vi "GUI_Shutdown.vi"(4 "error in":errorcluster) -> (0 "error out":errorcluster)   [LabVIEW 2015]
doc: "Monitors the manager globals, waiting for a complete shutdown"
panel:
  out "shutting down systems...":dbl(slide) scale=0.0..100.0
  in  "Listbox":i32(listbox)=8
  # "Systems are shutting down.  Mechanical systems are \nreturning to safe configurations. The program will \nterminate automatically when the shutdown is \ncomplete."
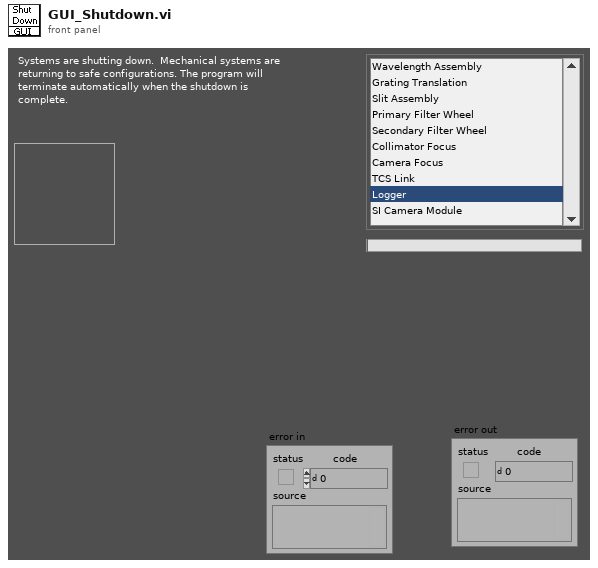
[diagram p1: front panel]
types:
  T1 = cluster{"WL Online":bool, "GT Online":bool, "Slit Online":bool, "F1 Online":bool, "F2 Online":bool, "Coll Online":bool, "CF Online":bool, "TCSLink Online":bool, "Logger Online":bool, "Apogee Online":bool, "TCPServer Online":bool}
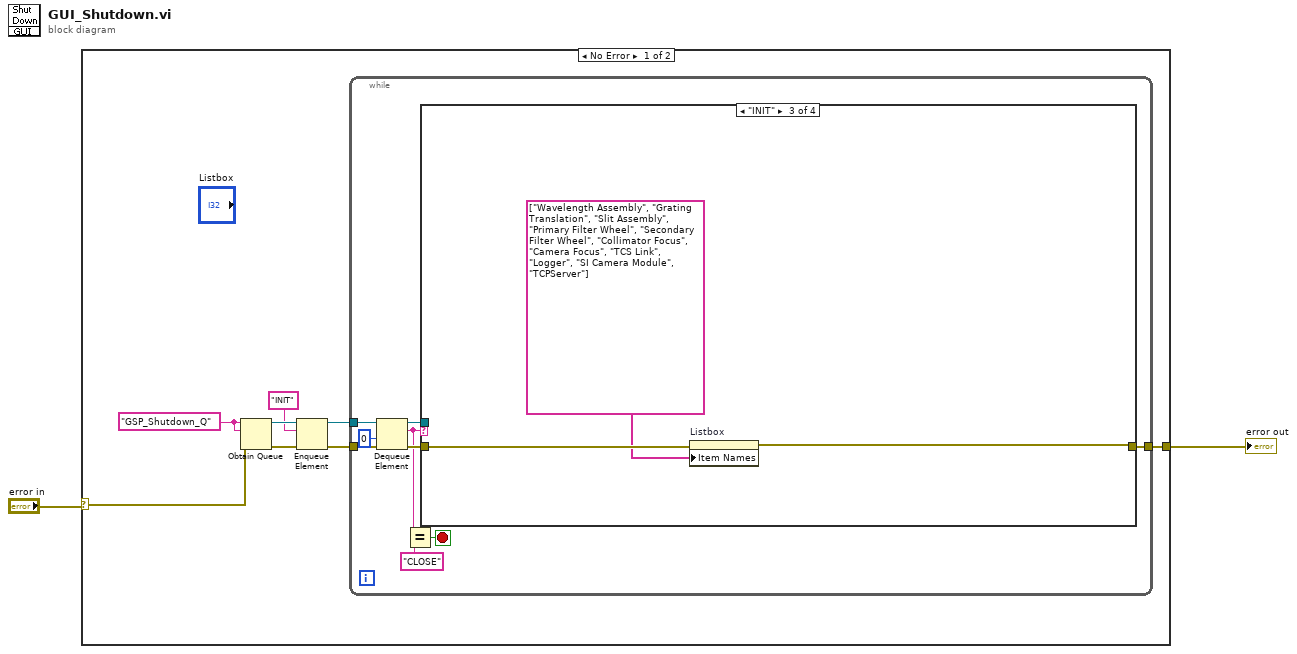
[diagram p0: block diagram]
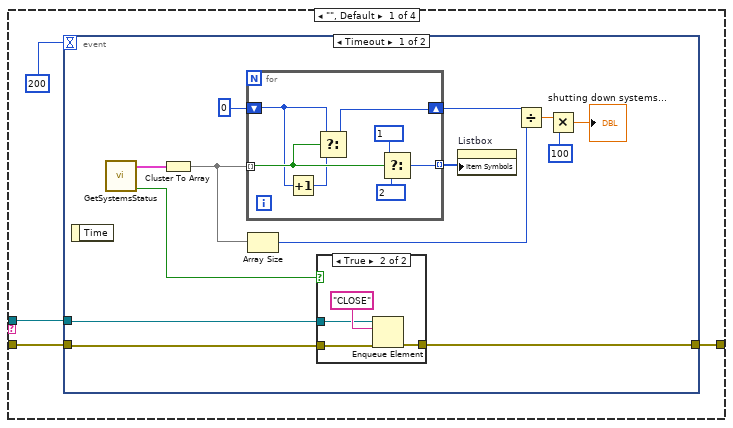
[diagram p2: hidden frame]
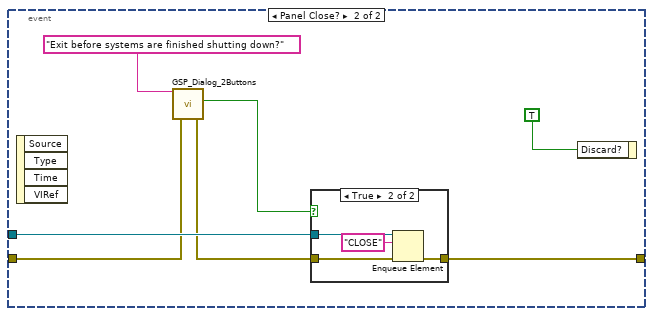
[diagram p4: hidden frame]
diagram:
  n1 = case shown="No Error" "error in" {
    selector: "error in" -> [w3 w66]
    tunnel: [w5 w66] -> w2
    frame No Error {
      w8 = "GSP_Shutdown_Q" ("name (unnamed)")
      n2 = Obtain Queue(name (unnamed)=w8, element data type=w8, error in (no error)=w3) -> (queue out=w9:refnum<queue>, error out=w10:errorcluster)  [unwired: 2 in, 1 out]
      n3 = Enqueue Element(queue=w9, element="INIT", error in (no error)=w10) -> (queue out=w7:refnum<queue>, error out=w6:errorcluster)  [unwired: 1 in, 1 out]
      n4 = while {
        tunnel: w7 -> [w19]
        tunnel: w6 -> [w18]
        tunnel: [w11] -> w5
        stop <- w13 stop-if-true
        n5 = Dequeue Element(queue=w19, timeout in ms (-1)=0, error in (no error)=w18) -> (queue out=w17:refnum<queue>, element=w15:string, error out=w16:errorcluster)  [unwired: 1 out]
        n6 = Equal?(x=w15, y="CLOSE") -> (x = y?=w13:bool)
        n7 = case shown="\"INIT\"" w15 {
          tunnel: w17 -> [w22 _ _ _]
          tunnel: w16 -> [w21 w61 w64 w65]
          tunnel: [w20 w61 w63 w65] -> w11
          frame "", Default {
            n8 = event shown="[0] Timeout" {
              selector: _ -> [_ _]
              dyn-events: _ -> [_ _]
              timeout: 200 -> [_ _]
              tunnel: w22 -> [w33 w53]
              tunnel: w21 -> [w36 w50]
              tunnel: [w35 w54] -> w20
              event Timeout {
                n9 = event-data() -> ()  [unwired: 1 in, 1 out]
                n10 = call "GetSystemsStatus.vi"() -> ("All systems offline?"=w32:bool, "Systems Online"=w31:T1)  [unwired: 4 in, 2 out]
                n11 = Cluster To Array(cluster=w31) -> (array=w29:bool[])
                n12 = for {
                  tunnel: [w43] -> w34 mode=indexing
                  tunnel: w29 -> [w40] mode=indexing
                  shift-right: [w37] -> w28
                  shift-left: 0 -> [w38]
                  n13 = Increment(x=w38) -> (x+1=w39:i32)
                  n14 = Select(t=w38, s=w40, f=w39) -> (s? t:f=w37:i32)
                  n15 = Select(t=1, s=w40, f=2) -> (s? t:f=w43:i32)
                }
                n16 = Array Size(array=w29) -> (size(s)=w26:i32)
                n17 = case shown="True" w32 {
                  tunnel: w36 -> [w44 w48]
                  tunnel: [w44 w47] -> w35
                  tunnel: w33 -> [_ w45]
                  frame False {
                  }
                  frame True {
                    n18 = Enqueue Element(queue=w45, element="CLOSE", error in (no error)=w48) -> (error out=w47:errorcluster)  [unwired: 1 in, 2 out]
                  }
                }
                n19 = property on="Listbox" class="LstBox (strict)"("Item Symbols"=w34) -> ()  [unwired: 2 in, 2 out]
                n20 = Divide(x=w28, y=w26) -> (x/y=w25:dbl)
                n21 = Multiply(x=w25, y=100) -> (x*y=→"shutting down systems...":dbl)
              }
              event Panel Close? {
                n22 = event-data() -> ()  [unwired: 1 in, 4 out]
                n23 = call "GSP_Dialog_2Buttons.vi"("error in (no error)"=w50, "Message"="Exit before systems are finished shutting down?" ("message")) -> ("error out"=w49:errorcluster, "OK Button?"=w51:bool)  [unwired: 4 in]
                n24 = case shown="True" w51 {
                  tunnel: [w56 w60] -> w54
                  tunnel: w49 -> [w56 w59]
                  tunnel: w53 -> [_ w58]
                  frame False {
                  }
                  frame True {
                    n25 = Enqueue Element(queue=w58, element="CLOSE", error in (no error)=w59) -> (error out=w60:errorcluster)  [unwired: 1 in, 2 out]
                  }
                }
                n26 = event-data("Discard?"=TRUE) -> ()  [unwired: 1 in, 1 out]
              }
            }
          }
          frame "CLOSE" {
          }
          frame "INIT" {
            n27 = property on="Listbox" class="LstBox (strict)"(error in=w64, "Item Names"=string[] ["Wavelength Assembly", "Grating Translation", "Slit Assembly", "Primary Filter Wheel", "Secondary Filter Wheel", "Collimator Focus", "Camera Focus", "TCS Link", "Logger", "SI Camera Module", "TCPServer"]) -> (error out=w63:errorcluster)  [unwired: 1 in, 1 out]
          }
          frame "READY" {
          }
        }
      }
    }
    frame Error {
    }
  }
  "error out" <- w2
